vi "color_sensor_akindu.vi"() -> ()   [LabVIEW 2022 SP3]
uses:
  <vilib>/DAQmx/create/channels.llb/DAQmx Create Channel (DO-Digital Output).vi
  <vilib>/DAQmx/write.llb/DAQmx Write (Digital Bool 1Line 1Point).vi
  <vilib>/DAQmx/create/channels.llb/DAQmx Create Channel (AI-Voltage-Basic).vi
  <vilib>/DAQmx/read.llb/DAQmx Read (Analog DBL 1Chan 1Samp).vi
panel:
  out "Array":dbl[](array[numeric])
  in  "physical channels":tag
  out "red 3":bool=TRUE
  out "red 2":bool=TRUE
  out "red":bool=TRUE
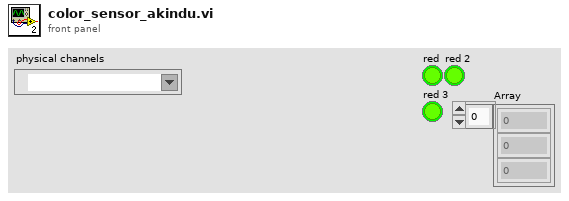
[diagram p1: front panel]
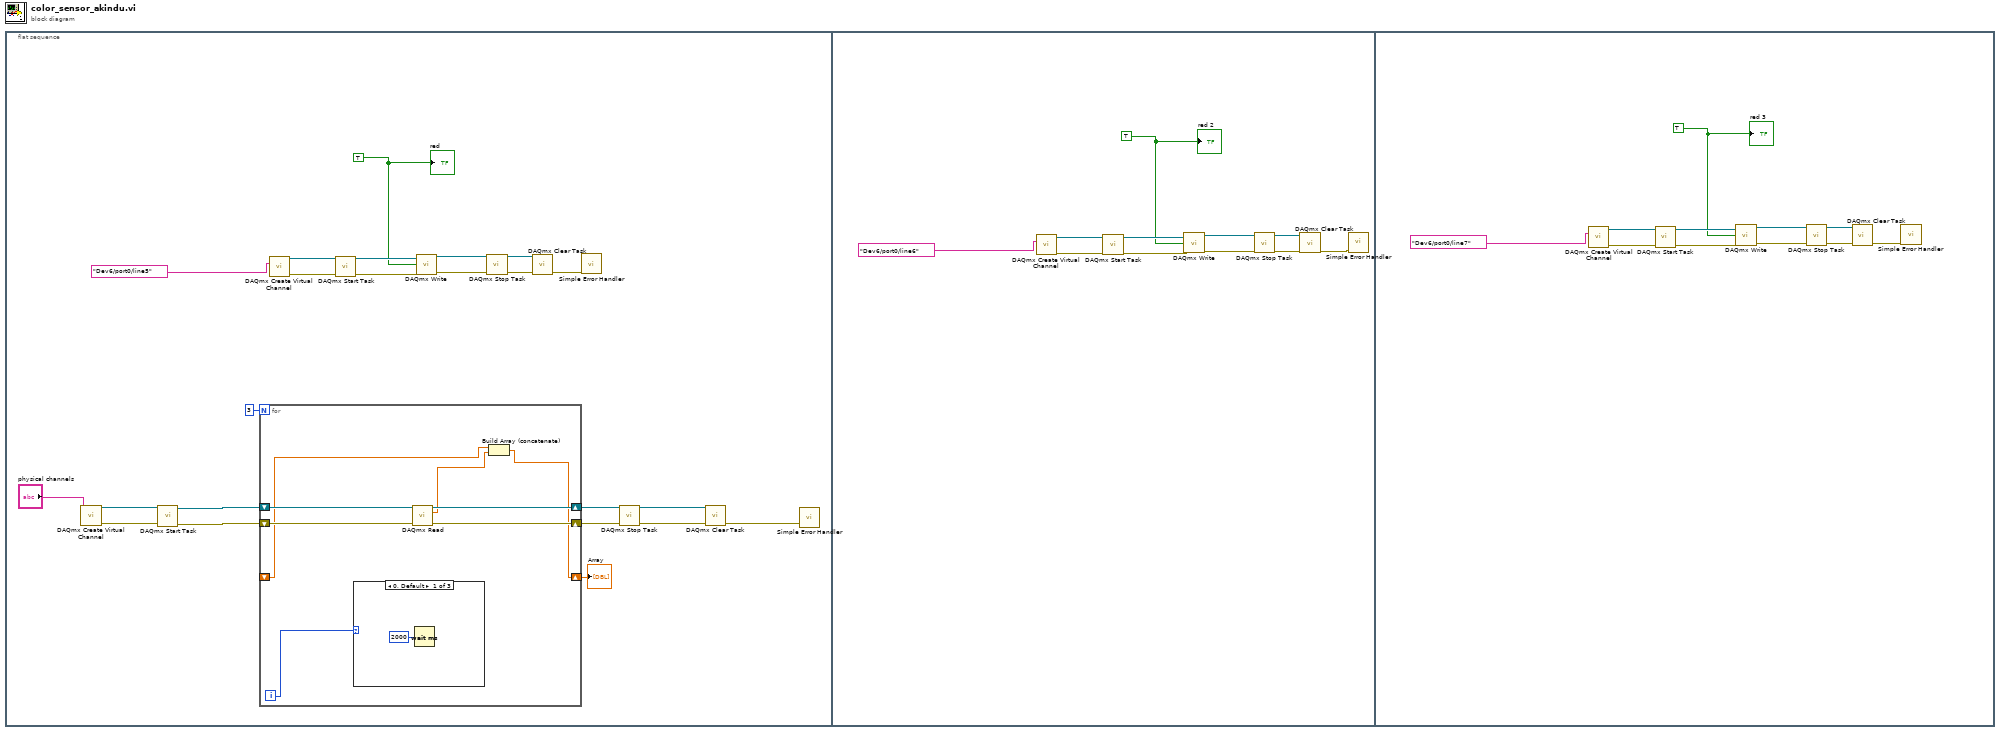
[diagram p0: block diagram]
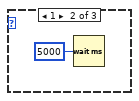
[diagram p2: hidden frame]
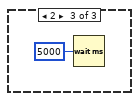
[diagram p3: hidden frame]
diagram:
  n1 = flat-sequence {
    frame #0 {
      w13 = TRUE ("data")
      n2 = call-poly <vilib>:"DAQmx Create Virtual Channel.vi"("physical channels"="physical channels") -> ("task out"=w11:refnum<k21>, "error out"=w12:errorcluster)  [unwired: 13 in]
      n3 = call <vilib>:"DAQmx Start Task.vi"("task/channels in"=w11, "error in"=w12) -> ("task out"=w6:refnum<k21>, "error out"=w5:errorcluster)  [unwired: 12 in]
      n4 = for {
        N: 3 -> [_]
        shift-right: [w29] -> w4
        shift-left: w6 -> [w31]
        shift-right: [w28] -> w3
        shift-left: w5 -> [w30]
        shift-right: [w24] -> w1
        shift-left: _ -> [w26]
        i -> [w27]
        n5 = case shown="0, Default" w27 {
          frame 0, Default {
            n6 = Wait (ms)(milliseconds to wait=u32 2000) -> ()  [unwired: 1 out]
          }
          frame 1 {
            n7 = Wait (ms)(milliseconds to wait=u32 5000) -> ()  [unwired: 1 out]
          }
          frame 2 {
            n8 = Wait (ms)(milliseconds to wait=u32 5000) -> ()  [unwired: 1 out]
          }
        }
        n9 = call-poly <vilib>:"DAQmx Read.vi"("task/channels in"=w31, "error in"=w30) -> ("task out"=w29:refnum<k21>, "data"=w25:dbl, "error out"=w28:errorcluster)  [unwired: 11 in]
        n10 = Build Array (concatenate)(w26, w25) -> (w24:dbl[])
      }
      "Array" <- w1
      n11 = call-poly <vilib>:"DAQmx Create Virtual Channel.vi"("lines"=tag "Dev6/port0/line5" ("Blue Channel")) -> ("task out"=w22:refnum<k21>, "error out"=w23:errorcluster)  [unwired: 13 in]
      n12 = call <vilib>:"DAQmx Start Task.vi"("task/channels in"=w22, "error in"=w23) -> ("task out"=w20:refnum<k21>, "error out"=w19:errorcluster)  [unwired: 12 in]
      n13 = call-poly <vilib>:"DAQmx Write.vi"("task/channels in"=w20, "data"=w13, "error in"=w19) -> ("task out"=w15:refnum<k21>, "error out"=w14:errorcluster)  [unwired: 10 in, 1 out]
      n14 = call <vilib>:"DAQmx Stop Task.vi"("task/channels in"=w15, "error in"=w14) -> ("task out"=w18:refnum<k21>, "error out"=w17:errorcluster)  [unwired: 12 in]
      n15 = call <vilib>:"DAQmx Clear Task.vi"("task in"=w18, "error in"=w17) -> ("error out"=w16:errorcluster)  [unwired: 13 in]
      n16 = call <vilib>:"Simple Error Handler.vi"("error in (no error)"=w16) -> ()  [unwired: 4 in, 5 out]
      n17 = call <vilib>:"DAQmx Stop Task.vi"("task/channels in"=w4, "error in"=w3) -> ("task out"=w10:refnum<k21>, "error out"=w9:errorcluster)  [unwired: 12 in]
      n18 = call <vilib>:"DAQmx Clear Task.vi"("task in"=w10, "error in"=w9) -> ("error out"=w8:errorcluster)  [unwired: 13 in]
      n19 = call <vilib>:"Simple Error Handler.vi"("error in (no error)"=w8) -> ()  [unwired: 4 in, 5 out]
      "red" <- w13
    }
    frame #1 {
      w35 = TRUE ("data")
      n20 = call-poly <vilib>:"DAQmx Create Virtual Channel.vi"("lines"=tag "Dev6/port0/line6" ("Blue Channel")) -> ("task out"=w44:refnum<k21>, "error out"=w45:errorcluster)  [unwired: 13 in]
      n21 = call <vilib>:"DAQmx Start Task.vi"("task/channels in"=w44, "error in"=w45) -> ("task out"=w42:refnum<k21>, "error out"=w41:errorcluster)  [unwired: 12 in]
      n22 = call-poly <vilib>:"DAQmx Write.vi"("task/channels in"=w42, "data"=w35, "error in"=w41) -> ("task out"=w37:refnum<k21>, "error out"=w36:errorcluster)  [unwired: 10 in, 1 out]
      n23 = call <vilib>:"DAQmx Stop Task.vi"("task/channels in"=w37, "error in"=w36) -> ("task out"=w40:refnum<k21>, "error out"=w39:errorcluster)  [unwired: 12 in]
      n24 = call <vilib>:"DAQmx Clear Task.vi"("task in"=w40, "error in"=w39) -> ("error out"=w38:errorcluster)  [unwired: 13 in]
      n25 = call <vilib>:"Simple Error Handler.vi"("error in (no error)"=w38) -> ()  [unwired: 4 in, 5 out]
      "red 2" <- w35
    }
    frame #2 {
      w46 = TRUE ("data")
      n26 = call-poly <vilib>:"DAQmx Create Virtual Channel.vi"("lines"=tag "Dev6/port0/line7" ("Blue Channel")) -> ("task out"=w55:refnum<k21>, "error out"=w56:errorcluster)  [unwired: 13 in]
      n27 = call <vilib>:"DAQmx Start Task.vi"("task/channels in"=w55, "error in"=w56) -> ("task out"=w53:refnum<k21>, "error out"=w52:errorcluster)  [unwired: 12 in]
      n28 = call-poly <vilib>:"DAQmx Write.vi"("task/channels in"=w53, "data"=w46, "error in"=w52) -> ("task out"=w48:refnum<k21>, "error out"=w47:errorcluster)  [unwired: 10 in, 1 out]
      n29 = call <vilib>:"DAQmx Stop Task.vi"("task/channels in"=w48, "error in"=w47) -> ("task out"=w51:refnum<k21>, "error out"=w50:errorcluster)  [unwired: 12 in]
      n30 = call <vilib>:"DAQmx Clear Task.vi"("task in"=w51, "error in"=w50) -> ("error out"=w49:errorcluster)  [unwired: 13 in]
      n31 = call <vilib>:"Simple Error Handler.vi"("error in (no error)"=w49) -> ()  [unwired: 4 in, 5 out]
      "red 3" <- w46
    }
  }
